vi "tqavgdata.vi"(0 "object in":refnum<class "212format_work.lvclass">, 1 "in":T2, 5 "error in (no error)":errorcluster) -> (14 "object out":refnum<class "212format_work.lvclass">, 15 "out":T1, 19 "error out":errorcluster)   [LabVIEW 2016, in "212format_work.lvclass"]
uses:
  212format_work.lvclass
  212format_work.lvclass/212format_work.ctl
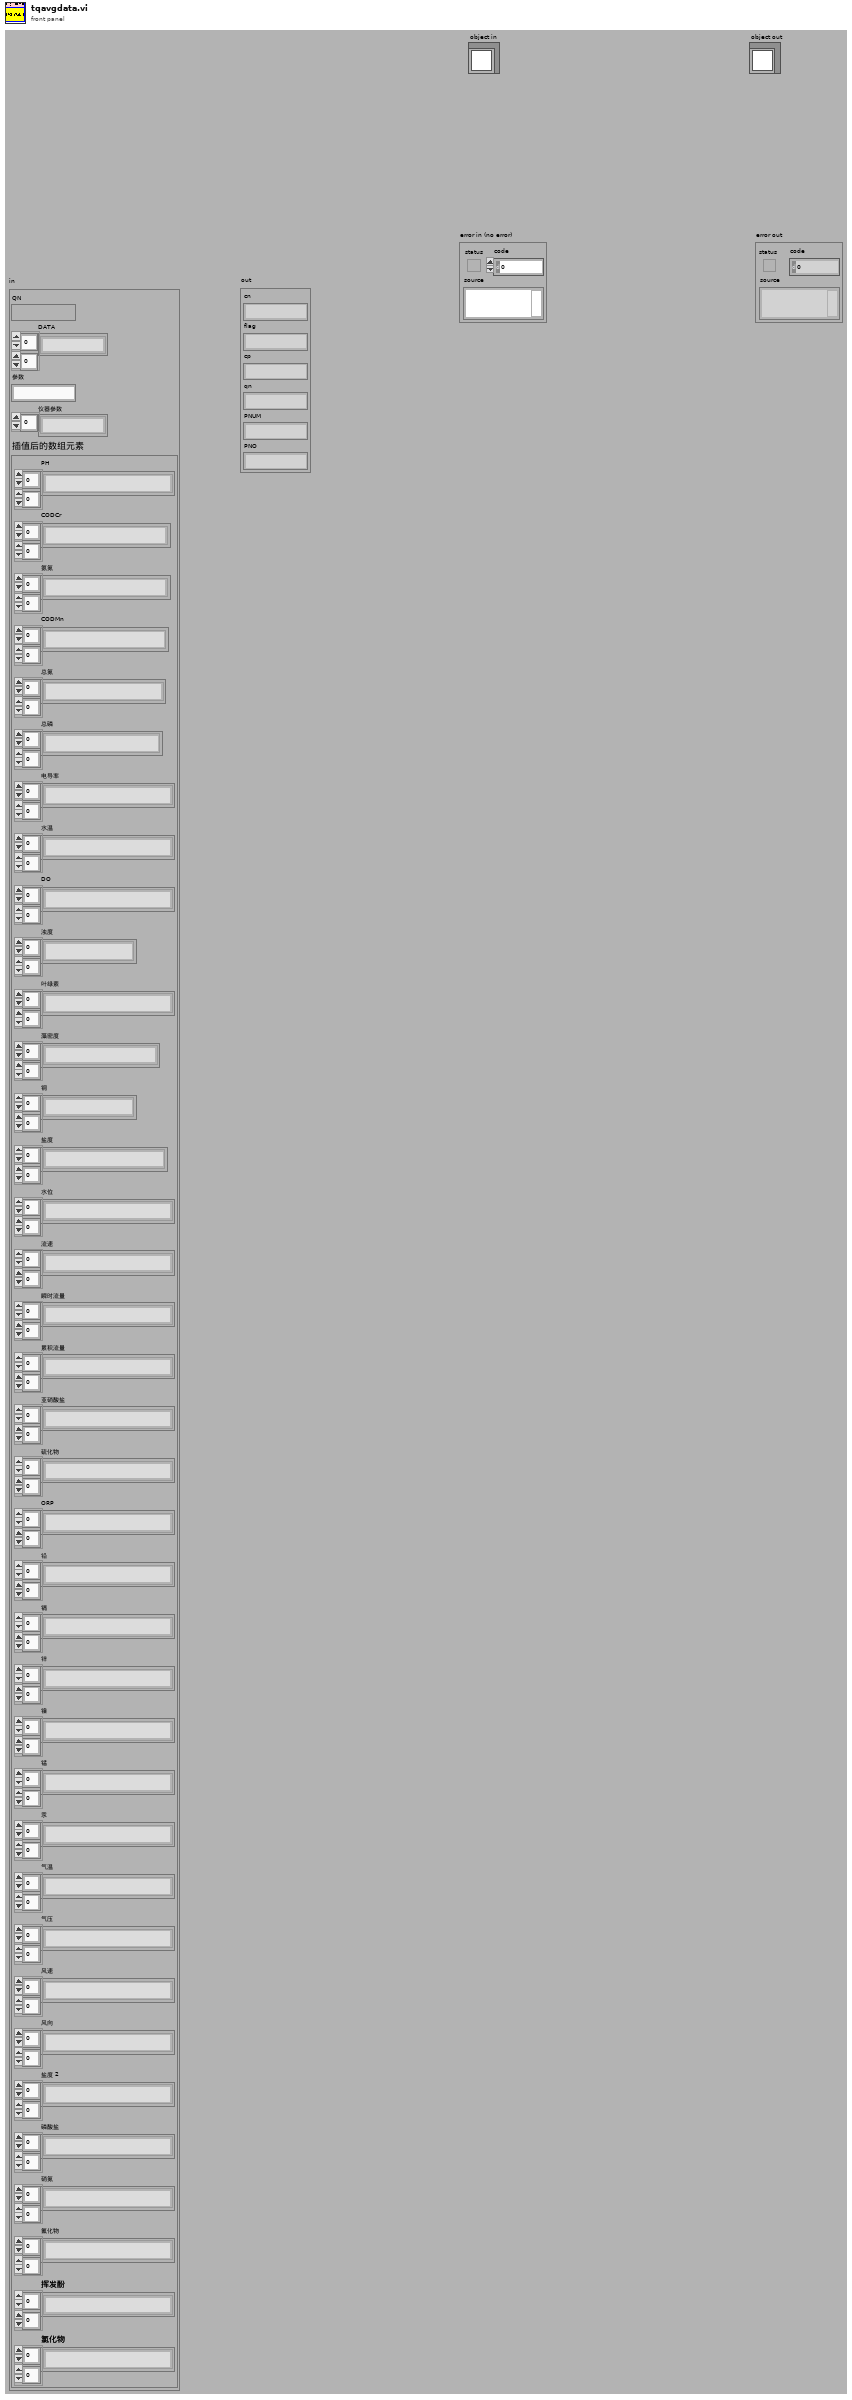
[diagram p1: front panel]
types:
  T1 = cluster{"cn":string, "flag":string, "cp":string, "qn":string, "PNUM":string, "PNO":string}
  T2 = cluster{"QN":string, "DATA":string[][], "参数":string, "仪器参数":string[], "插值后的数组元素":cluster{"PH":string[][], "CODCr":string[][], "氨氮":string[][], "CODMn":string[][], "总氮":string[][], "总磷":string[][], "电导率":string[][], "水温":string[][], "DO":string[][], "浊度":string[][], "叶绿素":string[][], "藻密度":string[][], "铜":string[][], "盐度":string[][], "水位":string[][], "流速":string[][], "瞬时流量":string[][], "累积流量":string[][], "亚硝酸盐":string[][], "硫化物":string[][], "ORP":string[][], "铅":string[][], "镉":string[][], "锌":string[][], "镍":string[][], "锰":string[][], "汞":string[][], "气温":string[][], "气压":string[][], "风速":string[][], "风向":string[][], "盐度 2":string[][], "磷酸盐":string[][], "硝氮":string[][], "氟化物":string[][], "挥发酚":string[][], "氯化物":string[][]}}
  T3 = enum16{"formattime", "formatminute", "formathour"}
  T4 = enum16{"小时数据", "实时数据", "平行样测试", "集成干预测试", "加标回收测试", "核查数据", "空白零点跨度数据", "提取小时数据", "提取实时数据", "操作日志", "仪器参数", "3090仪器参数", "提取仪器参数", "报警信息"}
  T5 = typedef "212format_work.lvclass/interdata控件.ctl" = cluster{"数据发送协议":enum16{"2005-212协议", "2017-212协议"}, "枚举":enum16{"返回请求应答", "上传数据", "返回执行结果"}, "系统编码ST":string, "主动上报数据中":bool, "数据组合发送":bool, "地表水/污染源":bool, "应用环境":enum16{"STD", "GB212"}}
  T6 = typedef "212format_work.lvclass/data控件.ctl" = cluster{"选择发送的参数":string, "插值后的数组元素":cluster{"PH":string[][], "CODCr":string[][], "氨氮":string[][], "CODMn":string[][], "总氮":string[][], "总磷":string[][], "电导率":string[][], "水温":string[][], "DO":string[][], "浊度":string[][], "叶绿素":string[][], "藻密度":string[][], "铜":string[][], "盐度":string[][], "水位":string[][], "流速":string[][], "瞬时流量":string[][], "累积流量":string[][], "亚硝酸盐":string[][], "硫化物":string[][], "ORP":string[][], "铅":string[][], "镉":string[][], "锌":string[][], "镍":string[][], "锰":string[][], "汞":string[][], "气温":string[][], "气压":string[][], "风速":string[][], "风向":string[][], "盐度 2":string[][], "磷酸盐":string[][], "硝氮":string[][], "氟化物":string[][], "挥发酚":string[][], "氯化物":string[][]}, "register values":u16[], "columns输出":string[], "环境参数":string[][], "仪器编码":string, "实时数据发送间隔":u32, "实时数据参数":string, "参数系数簇":cluster{"CODMn":dbl, "CODCr":dbl, "DO":dbl, "铜":dbl, "PH":dbl, "氨氮":dbl, "比电导率":dbl, "水温":dbl, "COD":dbl, "浊度":dbl, "总氮":dbl, "总磷":dbl, "叶绿素a":dbl, "藻密度":dbl, "水位":dbl, "流速":dbl, "瞬时流量":dbl, "累积流量":dbl, "亚硝酸盐":dbl, "硫化物":dbl, "ORP":dbl, "铅":dbl, "镉":dbl, "锌":dbl, "镍":dbl, "锰":dbl, "汞":dbl, "气温":dbl, "气压":dbl, "风速":dbl, "风向":dbl, "盐度":dbl, "磷酸盐":dbl, "硝氮":dbl, "氟化物":dbl, "挥发酚":dbl, "氯化物":dbl}, "因子编码簇":cluster{"CODMn":string, "CODCr":string, "DO":string, "铜":string, "PH":string, "氨氮":string, "比电导率":string, "水温":string, "COD":string, "浊度":string, "总氮":string, "总磷":string, "叶绿素a":string, "藻密度":string, "水位":string, "流速":string, "瞬时流量":string, "累积流量":string, "亚硝酸盐":string, "硫化物":string, "ORP":string, "铅":string, "镉":string, "锌":string, "镍":string, "锰":string, "汞":string, "气温":string, "气压":string, "风速":string, "风向":string, "盐度":string, "磷酸盐":string, "硝氮":string, "氟化物":string, "挥发酚":string, "氯化物":string}, "小时数据发送次数":i32, "读取试剂余量的值":u16[], "参数编码":string, "数据数组大小":i32, "总包数":i32, "当前包号":i32, "columns":string[], "剖面多参数":string[][], "分包标准":i32}
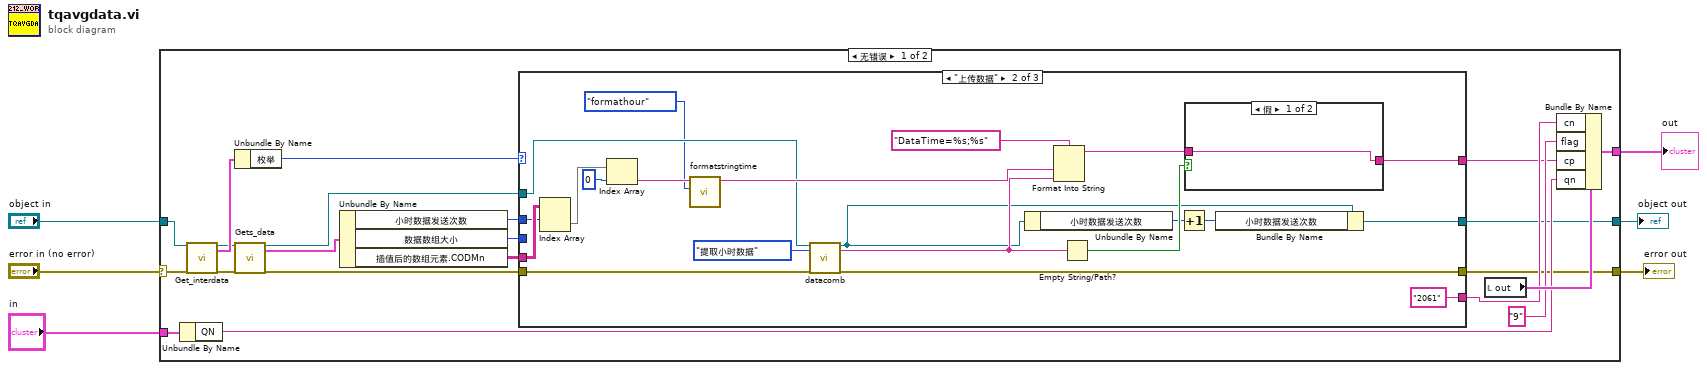
[diagram p0: block diagram]
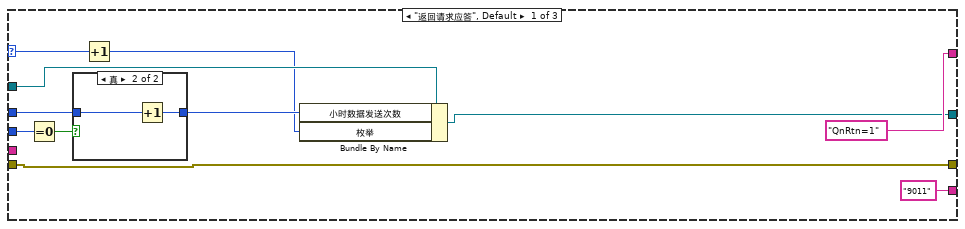
[diagram p2: hidden frame]
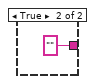
[diagram p4: hidden frame]
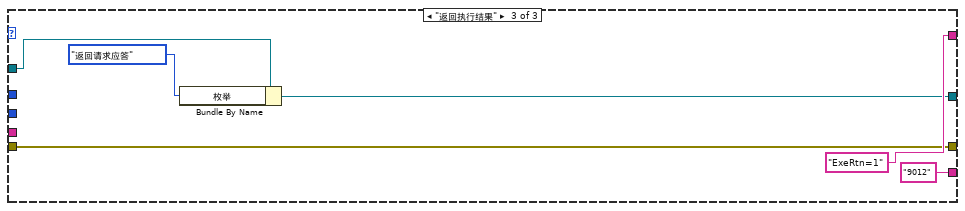
[diagram p5: hidden frame]
diagram:
  n1 = case shown="无错误" "error in (no error)" {
    selector: "error in (no error)" -> [w10 w72]
    tunnel: [w8 w72] -> w5
    tunnel: [w9 w71] -> w3
    tunnel: "object in" -> [w12 w71]
    tunnel: "in" -> [w11 _]
    tunnel: [w7 _] -> w1
    frame No Error {
      n2 = Unbundle By Name(w11) -> ("QN"=w26:string)
      n3 = call-dynamic "Get_interdata.vi"("object in"=w12, "error in (no error)"=w10) -> ("object out"=w20:refnum<class "212format_work.lvclass">, "interdata"=w22:T5, "error out"=w19:errorcluster)  [unwired: 15 in]
      n4 = Unbundle By Name(w22) -> ("枚举"=w21:enum16{"返回请求应答", "上传数据", "返回执行结果"})
      n5 = call-dynamic "Gets_data.vi"("object in"=w20, "error in (no error)"=w19) -> ("object out"=w15:refnum<class "212format_work.lvclass">, "data"=w18:T6, "error out"=w13:errorcluster)  [unwired: 15 in]
      n6 = Unbundle By Name(w18) -> ("小时数据发送次数"=w16:i32, "数据数组大小"=w17:i32, "插值后的数组元素.CODMn"=w14:string[][])
      n7 = case shown="\"上传数据\"" w21 {
        selector: w21 -> [w31 _ _]
        tunnel: ["9011" ("CN") "2061" ("CN") "9012" ("CN")] -> w25
        tunnel: ["QnRtn=1" w49 "ExeRtn=1"] -> w23
        tunnel: w15 -> [w36 w53 w68]
        tunnel: w17 -> [w35 _ _]
        tunnel: w16 -> [w33 w51 _]
        tunnel: [w29 w42 w66] -> w9
        tunnel: w14 -> [_ w52 _]
        tunnel: w13 -> [w28 w50 w65]
        tunnel: [w28 w48 w65] -> w8
        frame "返回请求应答", Default {
          n8 = Equal To 0?(x=w35) -> (x = 0?=w34:bool)
          n9 = case shown="真" w34 {
            tunnel: w33 -> [w39 w41]
            tunnel: [w39 w40] -> w32
            frame False {
            }
            frame True {
              n10 = Increment(x=w41) -> (x+1=w40:i32)
            }
          }
          n11 = Increment(x=w31) -> (x+1=w30:enum16{"返回请求应答", "上传数据", "返回执行结果"})
          n12 = Bundle By Name(cluster=w36, "小时数据发送次数"=w32, "枚举"=w30) -> (w29:refnum<class "212format_work.lvclass">)
        }
        frame "上传数据" {
          n13 = Index Array(array=w52, index (row)=w51) -> (element=w60:string[])  [unwired: 1 in]
          n14 = Index Array(array=w60, index=0 ("索引")) -> (element=w58:string)
          n15 = call "formatstringtime.vi"("枚举"=T3."formathour", "字符串"=w58) -> ("result string"=w55:string)  [unwired: 9 in]
          n16 = call-dynamic "datacomb.vi"("object in"=w53, "枚举"=T4."提取小时数据", "error in (no error)"=w50) -> ("object out"=w43:refnum<class "212format_work.lvclass">, "字符串"=w54:string, "error out"=w48:errorcluster)  [unwired: 14 in]
          n17 = Unbundle By Name(w43) -> ("小时数据发送次数"=w45:i32)
          n18 = Format Into String(format string="DataTime=%s;%s", w55, w54) -> (resulting string=w46:string)  [unwired: 2 in, 1 out]
          n19 = Empty String/Path?(string/path=w54) -> (empty?=w56:bool)
          n20 = Increment(x=w45) -> (x+1=w44:i32)
          n21 = case shown="假" w56 {
            tunnel: [w63 ""] -> w49
            tunnel: w46 -> [w63 _]
            frame False {
            }
            frame True {
            }
          }
          n22 = Bundle By Name(cluster=w43, "小时数据发送次数"=w44) -> (w42:refnum<class "212format_work.lvclass">)
        }
        frame "返回执行结果" {
          n23 = Bundle By Name(cluster=w68, "枚举"=enum16{"返回请求应答", "上传数据", "返回执行结果"}."返回请求应答" ("interdata.枚举")) -> (w66:refnum<class "212format_work.lvclass">)
        }
      }
      n24 = local read "out"() -> (w27:T1)
      n25 = Bundle By Name(cluster=w27, "cn"=w25, "flag"="9" ("ST"), "cp"=w23, "qn"=w26) -> (w7:T1)
    }
    frame Error {
    }
  }
  "error out" <- w5
  "object out" <- w3
  "out" <- w1
